vi "g_VBAIMeasurements.vi"() -> ()   [LabVIEW 2014]
panel:
  out "ReadEnable":bool
  out "Probe_D_Y":dbl
  out "Pad_D_Y":dbl
  out "Probe_C_Y":dbl
  out "Probe_B_X":dbl
  out "Probe_A_X":dbl
  out "Pad_C_Y":dbl
  out "Pad_B_X":dbl
  out "Pad_A_X":dbl
  out "Y_DistCornerVsensRight":dbl
  out "YPos_VsensRight":dbl
  out "YPos_NIL":dbl
  out "X_DistCornerVsensRight":dbl
  out "XPos_VsensRight":dbl
  out "XPos_NIL":dbl
  # "Preliminary Alignment Measurements"
  # "Adjustment Measurements"
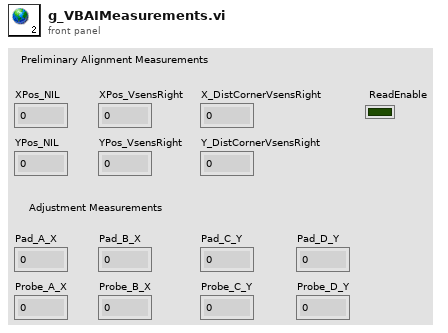
[diagram p1: front panel]
diagram:
